vi "USBTC08StreamingRun.vi"(8 "error in (no error)":errorcluster, 11 "Handle in":i16) -> (0 "error out":errorcluster, 2 "minimumIntervalMs":i32, 3 "Handle out":i16)   [LabVIEW 2009]
uses:
  usbtc08.dll
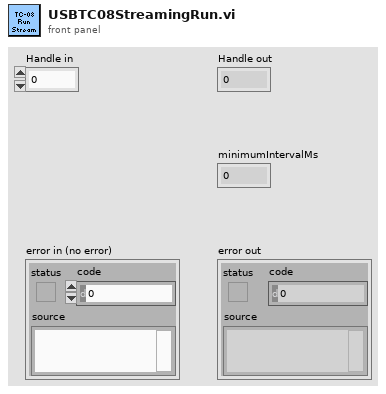
[diagram p1: front panel]
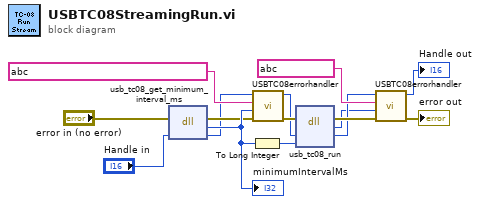
[diagram p0: block diagram]
diagram:
  n1 = dll-call lib="usbtc08.dll" fn="usb_tc08_get_minimum_interval_ms" ("Close unit")(error in="error in (no error)", "handle"="Handle in") -> (error out=w10:errorcluster, "return type"=w14:i32, "handle"=w2:i16)  [unwired: 2 in, 1 out]
  "minimumIntervalMs" <- w14
  n2 = To Long Integer(number=w14) -> (32bit integer=w9:i32)
  n3 = call "USBTC08errorhandler.vi"("error in (no error)"=w10, "Return"=w14, "API function"=string ?, "Handle in"=w2) -> ("error out"=w11:errorcluster, "Handle out"=w3:i16)  [unwired: 6 in]
  n4 = dll-call lib="usbtc08.dll" fn="usb_tc08_run" ("Close unit")(error in=w11, "handle"=w3, "interval"=w9) -> (error out=w12:errorcluster, "return type"=w4:i32, "handle"=w5:i16)  [unwired: 3 in, 1 out]
  n5 = call "USBTC08errorhandler.vi"("error in (no error)"=w12, "Return"=w4, "API function"=string ?, "Handle in"=w5) -> ("error out"=→"error out":errorcluster, "Handle out"=→"Handle out":i16)  [unwired: 6 in]
